vi "Load BMP SLM.vi"() -> (2 "double precision float":dbl[][](array[numeric]))   [LabVIEW 2014]
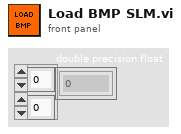
[diagram p1: front panel]
types:
  T1 = typedef "IMAQ Image.ctl" = refnum<image>
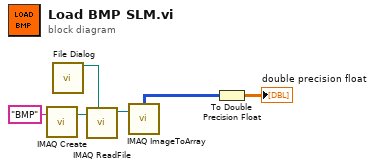
[diagram p0: block diagram]
diagram:
  n1 = call "IMAQ Create"("Image Name"="BMP") -> ("New Image"=w4:T1)  [unwired: 3 in, 2 out]
  n2 = call "File Dialog"() -> ("selected path"=w5:path)  [unwired: 7 in, 8 out]
  n3 = call "IMAQ ReadFile"("File Path"=w5, "Image"=w4) -> ("Image Out"=w6:T1)  [unwired: 3 in, 6 out]
  n4 = call "IMAQ ImageToArray"("Image"=w6) -> ("Image Pixels (U8)"=w2:u8[][])  [unwired: 2 in, 5 out]
  n5 = To Double Precision Float(number=w2) -> (double precision float=→"double precision float":dbl[][])
